vi "mxwScript_API_XMLTemplateName_AddTemplateRef.vi"(7 "templateRefType":T3, 8 "error in (no error)":errorcluster, 9 "terminalData":T2={"name"="", "termIsTag"=FALSE, "referencePosition"=enum."Middle"}, 10 "referencePosition":T1, 11 "absolutePath":string) -> (0 "error out":errorcluster, 3 "encoded absolutePath":string)   [LabVIEW 2020]
doc: "Add information to override the default method for locating the reference point on the block diagram during template drop."
uses:
  codeGenAPISupport.llb/cgAPI_mxwScript_DrpTmplt_TemplateRefType.ctl
  codeGenAPISupport.llb/cgAPI_mxwScript_DrpTmplt_TerminalData.ctl
  codeGenAPISupport.llb/cgAPI_mxwScript_DrpTmplt_ReferencePosition.ctl
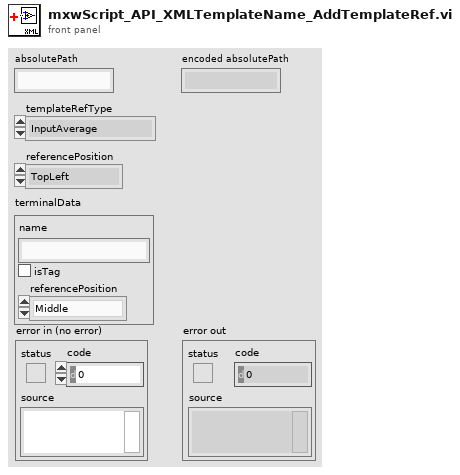
[diagram p1: front panel]
types:
  T1 = typedef "cgAPI_mxwScript_DrpTmplt_ReferencePosition.ctl" = enum16{"TopLeft", "Top", "TopRight", "Left", "Middle", "Right", "BottomLeft", "Bottom", "BottomRight"}
  T2 = typedef "cgAPI_mxwScript_DrpTmplt_TerminalData.ctl" = cluster{"name":string, "termIsTag":bool, "referencePosition":T1}
  T3 = typedef "cgAPI_mxwScript_DrpTmplt_TemplateRefType.ctl" = enum16{"InputAverage", "Absolute", "Terminal"}
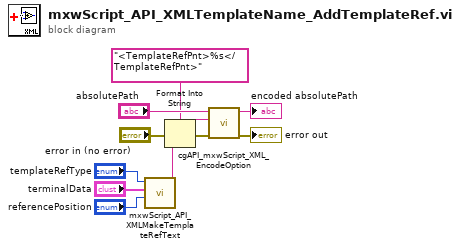
[diagram p0: block diagram]
diagram:
  n1 = call "mxwScript_API_XMLMakeTemplateRefText.vi"("referencePosition"="referencePosition", "terminalData"="terminalData", "templateRefType"="templateRefType") -> ("templateRefText"=w1:string)  [unwired: 8 out]
  n2 = Format Into String(format string="<TemplateRefPnt>%s</TemplateRefPnt>" ("control name"), error in="error in (no error)", w1) -> (resulting string=w6:string, error out=w8:errorcluster)  [unwired: 1 in]
  n3 = call "cgAPI_mxwScript_XML_EncodeOption.vi"("error in (no error)"=w8, "otherXML"=w6, "normalTextString"="absolutePath") -> ("error out"=→"error out":errorcluster, "encodedString"=→"encoded absolutePath":string)  [unwired: 7 out]
